vi "3Dlauncher.vi"(1 "dataFilePath":path, 2 "Data":string[][](array[string]), 3 "Template Filename":path, 4 "Channel Names":string[](array[string])) -> ()   [LabVIEW 2022 SP3]
uses:
  Anemometry/Anemometry Sub Vis/Controls/Group_Binning.ctl
  Anemometry/Anemometry Sub Vis/Data_plotting_vis/Results_plotter_Global.vi
panel:
  in  "Tab Control":enum32{"Page 1", "Page 2"}(tab)
  in  "Wind Direction":u16(ring) items=["Date Sortable", "Rig", "Run Command File", "Run Start Time", "Run Description", "Row Number", "Row Type", "Row Start (sec)", "Row Comment", "Timestamp", "Time In Row(s)", "Config", "Config Num", "Errata", "Omit", "WD", "WD.Pt", "WD.Pt.Cfg", "Point ID", "Point Row", "Legend0", "Downrange Distance (ft)", "Point Height Num", "Point Column", "Legend1", "- MeasuredVariables -----------", "-- VelocityStats --", "U_{dem} Nominal (m/s)", "U_{ref} (m/s)", "Uref ADAM (m/s)", "\\overline{U_{raw}} /U_{ref}", "U_{ref} ADAM /U_{ref}", "\\overline{U} (m/s)", "U corr (m/s)", "\\overline{V} (m/s)", "\\overline{W} (m/s)", "\\overline{|UV|} (m/s)", "\\overline{|UW|} (m/s)", "\\overline{|UVW|} (m/s)", "\\overline{\\theta} (deg)", "\\sigma^2(U) (m/s)^2", "\\sigma^2(V) (m/s)^2", "\\sigma^2(W) (m/s)^2", "\\sigma^2(|UV|) (m/s)^2", "\\sigma^2(|UW|) (m/s)^2", "\\sigma^2(|UVW|) (m/s)^2", "\\sigma^2(\\theta) (deg^2)", "u'v' (m^2/s^2)", "v'w' (m^2/s^2)", "u'w' (m^2/s^2)", "-- VelocityStatsEnd --", "-- QAstats --", "Omni meanPSU (V)", "Omni varPSU (V^2)", "Omni Cal Slope", "Omni Cal Intercept", "Temp (C)", "No Of Measurement Blocks", "No of Analogue Samples", "Flow Measurement Time", "Decimation", "AFRaw nGood perDecBlock", "AFGoodV nGood perDecBlock", "AFGoodVP nGood perDecBlock", "AFRaw nCone<58 deg", "AFRaw nCone<90 deg", "AFRaw Cone<58 deg", "AFRaw Cone<90 deg", "Run Messages", "-- QAstatsEnd --", "- MeasuredVariablesEnd -----------", "Max (ConeAngle) (deg)", "Valid AFReduction Fraction", "Valid Velocity Fraction", "Valid 5hpPressure Fraction", "- LocationsStart -------------", "Scale", "Probe Angle (deg)", "Row X 0", "X (mm)", "Y (mm)", "Z (mm)", "U_{ref} Z (mm)", "Metadata Motor X", "Metadata Motor Y", "Metadata Motor Z", "- LocationsEnd -------------", "- BLsetupBlock ------------", "BLS Trip[1] Ach(mm)", "BLS Trip[2] Ach(mm)", "BLS Spires[1] Ach(mm)", "BLS Spires[1]TipJoint Ach(mm)", "BLS Spires[1] Tips(mm)", "BLS Spires[2] Ach(mm)", "BLS Main[1] Ach(mm)", "BLS Main[2] Ach(mm)", "BLS Main[3] Ach(mm)", "BLS Boost[1] Ach(mm)", "BLS Boost[2] Ach(mm)", "BLS Boost[3] Ach(mm)", "Main Avg (mm)", "Boost Avg (mm)", "Spires[1] Total (mm)", "Ramp Request 0", "Ramp Request 1", "Ramp Request 2", "Ramp Request 3", "Ramp Request 4", "Ramp Request 5", "Ramp Request 6", "Ramp Request 7", "Ramp Request 8", "Ramp Request 9", "Ramp Request 10", "Ramp Request 11", "Ramp Request 12", "FORMATTED OUTPUT BELOW-THIS-------------", "Configuration", "Wind Direction (deg)", "BL Setup", "PointID", "Uref (m/s)", "Mean U /U_{ref}", "Mean V /U_{ref}", "Mean W /U_{ref}", "Mean |UV| /U_{ref}", "Mean |UW| /U_ref", "Mean |UVW| /U_ref", "Yaw (UV) (deg)", "TI (U) (/U)", "TI (U) (/|UV|)", "TI (V) (/|UV|)", "TI (W) (/|UW|)", "TI (|UV|) (/|UV|)", "TI (|UW|) (/|UW|)", "TI (|UVW|) (/|UVW|)", "TI Joint (%)", "Velocity Validation (percent)", "Raw Data Filename", "FORMATTED OUTPUT ABOVE-THIS---------------", "Current File", "Current Filepath", "Template File Used", "Seconds since 1st Jan", "Point Row Column", "Row Y", "X (in)", "Y (in)", "Z (in)", "STL name", "Coordinate System"]
  in  "STL":u16(ring) items=["Date Sortable", "Rig", "Run Command File", "Run Start Time", "Run Description", "Row Number", "Row Type", "Row Start (sec)", "Row Comment", "Timestamp", "Time In Row(s)", "Config", "Config Num", "Errata", "Omit", "WD", "WD.Pt", "WD.Pt.Cfg", "Point ID", "Point Row", "Legend0", "Downrange Distance (ft)", "Point Height Num", "Point Column", "Legend1", "- MeasuredVariables -----------", "-- VelocityStats --", "U_{dem} Nominal (m/s)", "U_{ref} (m/s)", "Uref ADAM (m/s)", "\\overline{U_{raw}} /U_{ref}", "U_{ref} ADAM /U_{ref}", "\\overline{U} (m/s)", "U corr (m/s)", "\\overline{V} (m/s)", "\\overline{W} (m/s)", "\\overline{|UV|} (m/s)", "\\overline{|UW|} (m/s)", "\\overline{|UVW|} (m/s)", "\\overline{\\theta} (deg)", "\\sigma^2(U) (m/s)^2", "\\sigma^2(V) (m/s)^2", "\\sigma^2(W) (m/s)^2", "\\sigma^2(|UV|) (m/s)^2", "\\sigma^2(|UW|) (m/s)^2", "\\sigma^2(|UVW|) (m/s)^2", "\\sigma^2(\\theta) (deg^2)", "u'v' (m^2/s^2)", "v'w' (m^2/s^2)", "u'w' (m^2/s^2)", "-- VelocityStatsEnd --", "-- QAstats --", "Omni meanPSU (V)", "Omni varPSU (V^2)", "Omni Cal Slope", "Omni Cal Intercept", "Temp (C)", "No Of Measurement Blocks", "No of Analogue Samples", "Flow Measurement Time", "Decimation", "AFRaw nGood perDecBlock", "AFGoodV nGood perDecBlock", "AFGoodVP nGood perDecBlock", "AFRaw nCone<58 deg", "AFRaw nCone<90 deg", "AFRaw Cone<58 deg", "AFRaw Cone<90 deg", "Run Messages", "-- QAstatsEnd --", "- MeasuredVariablesEnd -----------", "Max (ConeAngle) (deg)", "Valid AFReduction Fraction", "Valid Velocity Fraction", "Valid 5hpPressure Fraction", "- LocationsStart -------------", "Scale", "Probe Angle (deg)", "Row X 0", "X (mm)", "Y (mm)", "Z (mm)", "U_{ref} Z (mm)", "Metadata Motor X", "Metadata Motor Y", "Metadata Motor Z", "- LocationsEnd -------------", "- BLsetupBlock ------------", "BLS Trip[1] Ach(mm)", "BLS Trip[2] Ach(mm)", "BLS Spires[1] Ach(mm)", "BLS Spires[1]TipJoint Ach(mm)", "BLS Spires[1] Tips(mm)", "BLS Spires[2] Ach(mm)", "BLS Main[1] Ach(mm)", "BLS Main[2] Ach(mm)", "BLS Main[3] Ach(mm)", "BLS Boost[1] Ach(mm)", "BLS Boost[2] Ach(mm)", "BLS Boost[3] Ach(mm)", "Main Avg (mm)", "Boost Avg (mm)", "Spires[1] Total (mm)", "Ramp Request 0", "Ramp Request 1", "Ramp Request 2", "Ramp Request 3", "Ramp Request 4", "Ramp Request 5", "Ramp Request 6", "Ramp Request 7", "Ramp Request 8", "Ramp Request 9", "Ramp Request 10", "Ramp Request 11", "Ramp Request 12", "FORMATTED OUTPUT BELOW-THIS-------------", "Configuration", "Wind Direction (deg)", "BL Setup", "PointID", "Uref (m/s)", "Mean U /U_{ref}", "Mean V /U_{ref}", "Mean W /U_{ref}", "Mean |UV| /U_{ref}", "Mean |UW| /U_ref", "Mean |UVW| /U_ref", "Yaw (UV) (deg)", "TI (U) (/U)", "TI (U) (/|UV|)", "TI (V) (/|UV|)", "TI (W) (/|UW|)", "TI (|UV|) (/|UV|)", "TI (|UW|) (/|UW|)", "TI (|UVW|) (/|UVW|)", "TI Joint (%)", "Velocity Validation (percent)", "Raw Data Filename", "FORMATTED OUTPUT ABOVE-THIS---------------", "Current File", "Current Filepath", "Template File Used", "Seconds since 1st Jan", "Point Row Column", "Row Y", "X (in)", "Y (in)", "Z (in)", "STL name", "Coordinate System"]
  in  "OK Button":bool
  in  "vectorU":u16(ring) items=["Date Sortable", "Rig", "Run Command File", "Run Start Time", "Run Description", "Row Number", "Row Type", "Row Start (sec)", "Row Comment", "Timestamp", "Time In Row(s)", "Config", "Config Num", "Errata", "Omit", "WD", "WD.Pt", "WD.Pt.Cfg", "Point ID", "Point Row", "Legend0", "Downrange Distance (ft)", "Point Height Num", "Point Column", "Legend1", "- MeasuredVariables -----------", "-- VelocityStats --", "U_{dem} Nominal (m/s)", "U_{ref} (m/s)", "Uref ADAM (m/s)", "\\overline{U_{raw}} /U_{ref}", "U_{ref} ADAM /U_{ref}", "\\overline{U} (m/s)", "U corr (m/s)", "\\overline{V} (m/s)", "\\overline{W} (m/s)", "\\overline{|UV|} (m/s)", "\\overline{|UW|} (m/s)", "\\overline{|UVW|} (m/s)", "\\overline{\\theta} (deg)", "\\sigma^2(U) (m/s)^2", "\\sigma^2(V) (m/s)^2", "\\sigma^2(W) (m/s)^2", "\\sigma^2(|UV|) (m/s)^2", "\\sigma^2(|UW|) (m/s)^2", "\\sigma^2(|UVW|) (m/s)^2", "\\sigma^2(\\theta) (deg^2)", "u'v' (m^2/s^2)", "v'w' (m^2/s^2)", "u'w' (m^2/s^2)", "-- VelocityStatsEnd --", "-- QAstats --", "Omni meanPSU (V)", "Omni varPSU (V^2)", "Omni Cal Slope", "Omni Cal Intercept", "Temp (C)", "No Of Measurement Blocks", "No of Analogue Samples", "Flow Measurement Time", "Decimation", "AFRaw nGood perDecBlock", "AFGoodV nGood perDecBlock", "AFGoodVP nGood perDecBlock", "AFRaw nCone<58 deg", "AFRaw nCone<90 deg", "AFRaw Cone<58 deg", "AFRaw Cone<90 deg", "Run Messages", "-- QAstatsEnd --", "- MeasuredVariablesEnd -----------", "Max (ConeAngle) (deg)", "Valid AFReduction Fraction", "Valid Velocity Fraction", "Valid 5hpPressure Fraction", "- LocationsStart -------------", "Scale", "Probe Angle (deg)", "Row X 0", "X (mm)", "Y (mm)", "Z (mm)", "U_{ref} Z (mm)", "Metadata Motor X", "Metadata Motor Y", "Metadata Motor Z", "- LocationsEnd -------------", "- BLsetupBlock ------------", "BLS Trip[1] Ach(mm)", "BLS Trip[2] Ach(mm)", "BLS Spires[1] Ach(mm)", "BLS Spires[1]TipJoint Ach(mm)", "BLS Spires[1] Tips(mm)", "BLS Spires[2] Ach(mm)", "BLS Main[1] Ach(mm)", "BLS Main[2] Ach(mm)", "BLS Main[3] Ach(mm)", "BLS Boost[1] Ach(mm)", "BLS Boost[2] Ach(mm)", "BLS Boost[3] Ach(mm)", "Main Avg (mm)", "Boost Avg (mm)", "Spires[1] Total (mm)", "Ramp Request 0", "Ramp Request 1", "Ramp Request 2", "Ramp Request 3", "Ramp Request 4", "Ramp Request 5", "Ramp Request 6", "Ramp Request 7", "Ramp Request 8", "Ramp Request 9", "Ramp Request 10", "Ramp Request 11", "Ramp Request 12", "FORMATTED OUTPUT BELOW-THIS-------------", "Configuration", "Wind Direction (deg)", "BL Setup", "PointID", "Uref (m/s)", "Mean U /U_{ref}", "Mean V /U_{ref}", "Mean W /U_{ref}", "Mean |UV| /U_{ref}", "Mean |UW| /U_ref", "Mean |UVW| /U_ref", "Yaw (UV) (deg)", "TI (U) (/U)", "TI (U) (/|UV|)", "TI (V) (/|UV|)", "TI (W) (/|UW|)", "TI (|UV|) (/|UV|)", "TI (|UW|) (/|UW|)", "TI (|UVW|) (/|UVW|)", "TI Joint (%)", "Velocity Validation (percent)", "Raw Data Filename", "FORMATTED OUTPUT ABOVE-THIS---------------", "Current File", "Current Filepath", "Template File Used", "Seconds since 1st Jan", "Point Row Column", "Row Y", "X (in)", "Y (in)", "Z (in)", "STL name", "Coordinate System"]
  in  "vectorV":u16(ring) items=["Date Sortable", "Rig", "Run Command File", "Run Start Time", "Run Description", "Row Number", "Row Type", "Row Start (sec)", "Row Comment", "Timestamp", "Time In Row(s)", "Config", "Config Num", "Errata", "Omit", "WD", "WD.Pt", "WD.Pt.Cfg", "Point ID", "Point Row", "Legend0", "Downrange Distance (ft)", "Point Height Num", "Point Column", "Legend1", "- MeasuredVariables -----------", "-- VelocityStats --", "U_{dem} Nominal (m/s)", "U_{ref} (m/s)", "Uref ADAM (m/s)", "\\overline{U_{raw}} /U_{ref}", "U_{ref} ADAM /U_{ref}", "\\overline{U} (m/s)", "U corr (m/s)", "\\overline{V} (m/s)", "\\overline{W} (m/s)", "\\overline{|UV|} (m/s)", "\\overline{|UW|} (m/s)", "\\overline{|UVW|} (m/s)", "\\overline{\\theta} (deg)", "\\sigma^2(U) (m/s)^2", "\\sigma^2(V) (m/s)^2", "\\sigma^2(W) (m/s)^2", "\\sigma^2(|UV|) (m/s)^2", "\\sigma^2(|UW|) (m/s)^2", "\\sigma^2(|UVW|) (m/s)^2", "\\sigma^2(\\theta) (deg^2)", "u'v' (m^2/s^2)", "v'w' (m^2/s^2)", "u'w' (m^2/s^2)", "-- VelocityStatsEnd --", "-- QAstats --", "Omni meanPSU (V)", "Omni varPSU (V^2)", "Omni Cal Slope", "Omni Cal Intercept", "Temp (C)", "No Of Measurement Blocks", "No of Analogue Samples", "Flow Measurement Time", "Decimation", "AFRaw nGood perDecBlock", "AFGoodV nGood perDecBlock", "AFGoodVP nGood perDecBlock", "AFRaw nCone<58 deg", "AFRaw nCone<90 deg", "AFRaw Cone<58 deg", "AFRaw Cone<90 deg", "Run Messages", "-- QAstatsEnd --", "- MeasuredVariablesEnd -----------", "Max (ConeAngle) (deg)", "Valid AFReduction Fraction", "Valid Velocity Fraction", "Valid 5hpPressure Fraction", "- LocationsStart -------------", "Scale", "Probe Angle (deg)", "Row X 0", "X (mm)", "Y (mm)", "Z (mm)", "U_{ref} Z (mm)", "Metadata Motor X", "Metadata Motor Y", "Metadata Motor Z", "- LocationsEnd -------------", "- BLsetupBlock ------------", "BLS Trip[1] Ach(mm)", "BLS Trip[2] Ach(mm)", "BLS Spires[1] Ach(mm)", "BLS Spires[1]TipJoint Ach(mm)", "BLS Spires[1] Tips(mm)", "BLS Spires[2] Ach(mm)", "BLS Main[1] Ach(mm)", "BLS Main[2] Ach(mm)", "BLS Main[3] Ach(mm)", "BLS Boost[1] Ach(mm)", "BLS Boost[2] Ach(mm)", "BLS Boost[3] Ach(mm)", "Main Avg (mm)", "Boost Avg (mm)", "Spires[1] Total (mm)", "Ramp Request 0", "Ramp Request 1", "Ramp Request 2", "Ramp Request 3", "Ramp Request 4", "Ramp Request 5", "Ramp Request 6", "Ramp Request 7", "Ramp Request 8", "Ramp Request 9", "Ramp Request 10", "Ramp Request 11", "Ramp Request 12", "FORMATTED OUTPUT BELOW-THIS-------------", "Configuration", "Wind Direction (deg)", "BL Setup", "PointID", "Uref (m/s)", "Mean U /U_{ref}", "Mean V /U_{ref}", "Mean W /U_{ref}", "Mean |UV| /U_{ref}", "Mean |UW| /U_ref", "Mean |UVW| /U_ref", "Yaw (UV) (deg)", "TI (U) (/U)", "TI (U) (/|UV|)", "TI (V) (/|UV|)", "TI (W) (/|UW|)", "TI (|UV|) (/|UV|)", "TI (|UW|) (/|UW|)", "TI (|UVW|) (/|UVW|)", "TI Joint (%)", "Velocity Validation (percent)", "Raw Data Filename", "FORMATTED OUTPUT ABOVE-THIS---------------", "Current File", "Current Filepath", "Template File Used", "Seconds since 1st Jan", "Point Row Column", "Row Y", "X (in)", "Y (in)", "Z (in)", "STL name", "Coordinate System"]
  in  "vectorW":u16(ring) items=["Date Sortable", "Rig", "Run Command File", "Run Start Time", "Run Description", "Row Number", "Row Type", "Row Start (sec)", "Row Comment", "Timestamp", "Time In Row(s)", "Config", "Config Num", "Errata", "Omit", "WD", "WD.Pt", "WD.Pt.Cfg", "Point ID", "Point Row", "Legend0", "Downrange Distance (ft)", "Point Height Num", "Point Column", "Legend1", "- MeasuredVariables -----------", "-- VelocityStats --", "U_{dem} Nominal (m/s)", "U_{ref} (m/s)", "Uref ADAM (m/s)", "\\overline{U_{raw}} /U_{ref}", "U_{ref} ADAM /U_{ref}", "\\overline{U} (m/s)", "U corr (m/s)", "\\overline{V} (m/s)", "\\overline{W} (m/s)", "\\overline{|UV|} (m/s)", "\\overline{|UW|} (m/s)", "\\overline{|UVW|} (m/s)", "\\overline{\\theta} (deg)", "\\sigma^2(U) (m/s)^2", "\\sigma^2(V) (m/s)^2", "\\sigma^2(W) (m/s)^2", "\\sigma^2(|UV|) (m/s)^2", "\\sigma^2(|UW|) (m/s)^2", "\\sigma^2(|UVW|) (m/s)^2", "\\sigma^2(\\theta) (deg^2)", "u'v' (m^2/s^2)", "v'w' (m^2/s^2)", "u'w' (m^2/s^2)", "-- VelocityStatsEnd --", "-- QAstats --", "Omni meanPSU (V)", "Omni varPSU (V^2)", "Omni Cal Slope", "Omni Cal Intercept", "Temp (C)", "No Of Measurement Blocks", "No of Analogue Samples", "Flow Measurement Time", "Decimation", "AFRaw nGood perDecBlock", "AFGoodV nGood perDecBlock", "AFGoodVP nGood perDecBlock", "AFRaw nCone<58 deg", "AFRaw nCone<90 deg", "AFRaw Cone<58 deg", "AFRaw Cone<90 deg", "Run Messages", "-- QAstatsEnd --", "- MeasuredVariablesEnd -----------", "Max (ConeAngle) (deg)", "Valid AFReduction Fraction", "Valid Velocity Fraction", "Valid 5hpPressure Fraction", "- LocationsStart -------------", "Scale", "Probe Angle (deg)", "Row X 0", "X (mm)", "Y (mm)", "Z (mm)", "U_{ref} Z (mm)", "Metadata Motor X", "Metadata Motor Y", "Metadata Motor Z", "- LocationsEnd -------------", "- BLsetupBlock ------------", "BLS Trip[1] Ach(mm)", "BLS Trip[2] Ach(mm)", "BLS Spires[1] Ach(mm)", "BLS Spires[1]TipJoint Ach(mm)", "BLS Spires[1] Tips(mm)", "BLS Spires[2] Ach(mm)", "BLS Main[1] Ach(mm)", "BLS Main[2] Ach(mm)", "BLS Main[3] Ach(mm)", "BLS Boost[1] Ach(mm)", "BLS Boost[2] Ach(mm)", "BLS Boost[3] Ach(mm)", "Main Avg (mm)", "Boost Avg (mm)", "Spires[1] Total (mm)", "Ramp Request 0", "Ramp Request 1", "Ramp Request 2", "Ramp Request 3", "Ramp Request 4", "Ramp Request 5", "Ramp Request 6", "Ramp Request 7", "Ramp Request 8", "Ramp Request 9", "Ramp Request 10", "Ramp Request 11", "Ramp Request 12", "FORMATTED OUTPUT BELOW-THIS-------------", "Configuration", "Wind Direction (deg)", "BL Setup", "PointID", "Uref (m/s)", "Mean U /U_{ref}", "Mean V /U_{ref}", "Mean W /U_{ref}", "Mean |UV| /U_{ref}", "Mean |UW| /U_ref", "Mean |UVW| /U_ref", "Yaw (UV) (deg)", "TI (U) (/U)", "TI (U) (/|UV|)", "TI (V) (/|UV|)", "TI (W) (/|UW|)", "TI (|UV|) (/|UV|)", "TI (|UW|) (/|UW|)", "TI (|UVW|) (/|UVW|)", "TI Joint (%)", "Velocity Validation (percent)", "Raw Data Filename", "FORMATTED OUTPUT ABOVE-THIS---------------", "Current File", "Current Filepath", "Template File Used", "Seconds since 1st Jan", "Point Row Column", "Row Y", "X (in)", "Y (in)", "Z (in)", "STL name", "Coordinate System"]
  in  "Scalar":u16(ring) items=["Date Sortable", "Rig", "Run Command File", "Run Start Time", "Run Description", "Row Number", "Row Type", "Row Start (sec)", "Row Comment", "Timestamp", "Time In Row(s)", "Config", "Config Num", "Errata", "Omit", "WD", "WD.Pt", "WD.Pt.Cfg", "Point ID", "Point Row", "Legend0", "Downrange Distance (ft)", "Point Height Num", "Point Column", "Legend1", "- MeasuredVariables -----------", "-- VelocityStats --", "U_{dem} Nominal (m/s)", "U_{ref} (m/s)", "Uref ADAM (m/s)", "\\overline{U_{raw}} /U_{ref}", "U_{ref} ADAM /U_{ref}", "\\overline{U} (m/s)", "U corr (m/s)", "\\overline{V} (m/s)", "\\overline{W} (m/s)", "\\overline{|UV|} (m/s)", "\\overline{|UW|} (m/s)", "\\overline{|UVW|} (m/s)", "\\overline{\\theta} (deg)", "\\sigma^2(U) (m/s)^2", "\\sigma^2(V) (m/s)^2", "\\sigma^2(W) (m/s)^2", "\\sigma^2(|UV|) (m/s)^2", "\\sigma^2(|UW|) (m/s)^2", "\\sigma^2(|UVW|) (m/s)^2", "\\sigma^2(\\theta) (deg^2)", "u'v' (m^2/s^2)", "v'w' (m^2/s^2)", "u'w' (m^2/s^2)", "-- VelocityStatsEnd --", "-- QAstats --", "Omni meanPSU (V)", "Omni varPSU (V^2)", "Omni Cal Slope", "Omni Cal Intercept", "Temp (C)", "No Of Measurement Blocks", "No of Analogue Samples", "Flow Measurement Time", "Decimation", "AFRaw nGood perDecBlock", "AFGoodV nGood perDecBlock", "AFGoodVP nGood perDecBlock", "AFRaw nCone<58 deg", "AFRaw nCone<90 deg", "AFRaw Cone<58 deg", "AFRaw Cone<90 deg", "Run Messages", "-- QAstatsEnd --", "- MeasuredVariablesEnd -----------", "Max (ConeAngle) (deg)", "Valid AFReduction Fraction", "Valid Velocity Fraction", "Valid 5hpPressure Fraction", "- LocationsStart -------------", "Scale", "Probe Angle (deg)", "Row X 0", "X (mm)", "Y (mm)", "Z (mm)", "U_{ref} Z (mm)", "Metadata Motor X", "Metadata Motor Y", "Metadata Motor Z", "- LocationsEnd -------------", "- BLsetupBlock ------------", "BLS Trip[1] Ach(mm)", "BLS Trip[2] Ach(mm)", "BLS Spires[1] Ach(mm)", "BLS Spires[1]TipJoint Ach(mm)", "BLS Spires[1] Tips(mm)", "BLS Spires[2] Ach(mm)", "BLS Main[1] Ach(mm)", "BLS Main[2] Ach(mm)", "BLS Main[3] Ach(mm)", "BLS Boost[1] Ach(mm)", "BLS Boost[2] Ach(mm)", "BLS Boost[3] Ach(mm)", "Main Avg (mm)", "Boost Avg (mm)", "Spires[1] Total (mm)", "Ramp Request 0", "Ramp Request 1", "Ramp Request 2", "Ramp Request 3", "Ramp Request 4", "Ramp Request 5", "Ramp Request 6", "Ramp Request 7", "Ramp Request 8", "Ramp Request 9", "Ramp Request 10", "Ramp Request 11", "Ramp Request 12", "FORMATTED OUTPUT BELOW-THIS-------------", "Configuration", "Wind Direction (deg)", "BL Setup", "PointID", "Uref (m/s)", "Mean U /U_{ref}", "Mean V /U_{ref}", "Mean W /U_{ref}", "Mean |UV| /U_{ref}", "Mean |UW| /U_ref", "Mean |UVW| /U_ref", "Yaw (UV) (deg)", "TI (U) (/U)", "TI (U) (/|UV|)", "TI (V) (/|UV|)", "TI (W) (/|UW|)", "TI (|UV|) (/|UV|)", "TI (|UW|) (/|UW|)", "TI (|UVW|) (/|UVW|)", "TI Joint (%)", "Velocity Validation (percent)", "Raw Data Filename", "FORMATTED OUTPUT ABOVE-THIS---------------", "Current File", "Current Filepath", "Template File Used", "Seconds since 1st Jan", "Point Row Column", "Row Y", "X (in)", "Y (in)", "Z (in)", "STL name", "Coordinate System"]
  in  "Location X":u16(ring) items=["Date Sortable", "Rig", "Run Command File", "Run Start Time", "Run Description", "Row Number", "Row Type", "Row Start (sec)", "Row Comment", "Timestamp", "Time In Row(s)", "Config", "Config Num", "Errata", "Omit", "WD", "WD.Pt", "WD.Pt.Cfg", "Point ID", "Point Row", "Legend0", "Downrange Distance (ft)", "Point Height Num", "Point Column", "Legend1", "- MeasuredVariables -----------", "-- VelocityStats --", "U_{dem} Nominal (m/s)", "U_{ref} (m/s)", "Uref ADAM (m/s)", "\\overline{U_{raw}} /U_{ref}", "U_{ref} ADAM /U_{ref}", "\\overline{U} (m/s)", "U corr (m/s)", "\\overline{V} (m/s)", "\\overline{W} (m/s)", "\\overline{|UV|} (m/s)", "\\overline{|UW|} (m/s)", "\\overline{|UVW|} (m/s)", "\\overline{\\theta} (deg)", "\\sigma^2(U) (m/s)^2", "\\sigma^2(V) (m/s)^2", "\\sigma^2(W) (m/s)^2", "\\sigma^2(|UV|) (m/s)^2", "\\sigma^2(|UW|) (m/s)^2", "\\sigma^2(|UVW|) (m/s)^2", "\\sigma^2(\\theta) (deg^2)", "u'v' (m^2/s^2)", "v'w' (m^2/s^2)", "u'w' (m^2/s^2)", "-- VelocityStatsEnd --", "-- QAstats --", "Omni meanPSU (V)", "Omni varPSU (V^2)", "Omni Cal Slope", "Omni Cal Intercept", "Temp (C)", "No Of Measurement Blocks", "No of Analogue Samples", "Flow Measurement Time", "Decimation", "AFRaw nGood perDecBlock", "AFGoodV nGood perDecBlock", "AFGoodVP nGood perDecBlock", "AFRaw nCone<58 deg", "AFRaw nCone<90 deg", "AFRaw Cone<58 deg", "AFRaw Cone<90 deg", "Run Messages", "-- QAstatsEnd --", "- MeasuredVariablesEnd -----------", "Max (ConeAngle) (deg)", "Valid AFReduction Fraction", "Valid Velocity Fraction", "Valid 5hpPressure Fraction", "- LocationsStart -------------", "Scale", "Probe Angle (deg)", "Row X 0", "X (mm)", "Y (mm)", "Z (mm)", "U_{ref} Z (mm)", "Metadata Motor X", "Metadata Motor Y", "Metadata Motor Z", "- LocationsEnd -------------", "- BLsetupBlock ------------", "BLS Trip[1] Ach(mm)", "BLS Trip[2] Ach(mm)", "BLS Spires[1] Ach(mm)", "BLS Spires[1]TipJoint Ach(mm)", "BLS Spires[1] Tips(mm)", "BLS Spires[2] Ach(mm)", "BLS Main[1] Ach(mm)", "BLS Main[2] Ach(mm)", "BLS Main[3] Ach(mm)", "BLS Boost[1] Ach(mm)", "BLS Boost[2] Ach(mm)", "BLS Boost[3] Ach(mm)", "Main Avg (mm)", "Boost Avg (mm)", "Spires[1] Total (mm)", "Ramp Request 0", "Ramp Request 1", "Ramp Request 2", "Ramp Request 3", "Ramp Request 4", "Ramp Request 5", "Ramp Request 6", "Ramp Request 7", "Ramp Request 8", "Ramp Request 9", "Ramp Request 10", "Ramp Request 11", "Ramp Request 12", "FORMATTED OUTPUT BELOW-THIS-------------", "Configuration", "Wind Direction (deg)", "BL Setup", "PointID", "Uref (m/s)", "Mean U /U_{ref}", "Mean V /U_{ref}", "Mean W /U_{ref}", "Mean |UV| /U_{ref}", "Mean |UW| /U_ref", "Mean |UVW| /U_ref", "Yaw (UV) (deg)", "TI (U) (/U)", "TI (U) (/|UV|)", "TI (V) (/|UV|)", "TI (W) (/|UW|)", "TI (|UV|) (/|UV|)", "TI (|UW|) (/|UW|)", "TI (|UVW|) (/|UVW|)", "TI Joint (%)", "Velocity Validation (percent)", "Raw Data Filename", "FORMATTED OUTPUT ABOVE-THIS---------------", "Current File", "Current Filepath", "Template File Used", "Seconds since 1st Jan", "Point Row Column", "Row Y", "X (in)", "Y (in)", "Z (in)", "STL name", "Coordinate System"]
  in  "Location Y":u16(ring) items=["Date Sortable", "Rig", "Run Command File", "Run Start Time", "Run Description", "Row Number", "Row Type", "Row Start (sec)", "Row Comment", "Timestamp", "Time In Row(s)", "Config", "Config Num", "Errata", "Omit", "WD", "WD.Pt", "WD.Pt.Cfg", "Point ID", "Point Row", "Legend0", "Downrange Distance (ft)", "Point Height Num", "Point Column", "Legend1", "- MeasuredVariables -----------", "-- VelocityStats --", "U_{dem} Nominal (m/s)", "U_{ref} (m/s)", "Uref ADAM (m/s)", "\\overline{U_{raw}} /U_{ref}", "U_{ref} ADAM /U_{ref}", "\\overline{U} (m/s)", "U corr (m/s)", "\\overline{V} (m/s)", "\\overline{W} (m/s)", "\\overline{|UV|} (m/s)", "\\overline{|UW|} (m/s)", "\\overline{|UVW|} (m/s)", "\\overline{\\theta} (deg)", "\\sigma^2(U) (m/s)^2", "\\sigma^2(V) (m/s)^2", "\\sigma^2(W) (m/s)^2", "\\sigma^2(|UV|) (m/s)^2", "\\sigma^2(|UW|) (m/s)^2", "\\sigma^2(|UVW|) (m/s)^2", "\\sigma^2(\\theta) (deg^2)", "u'v' (m^2/s^2)", "v'w' (m^2/s^2)", "u'w' (m^2/s^2)", "-- VelocityStatsEnd --", "-- QAstats --", "Omni meanPSU (V)", "Omni varPSU (V^2)", "Omni Cal Slope", "Omni Cal Intercept", "Temp (C)", "No Of Measurement Blocks", "No of Analogue Samples", "Flow Measurement Time", "Decimation", "AFRaw nGood perDecBlock", "AFGoodV nGood perDecBlock", "AFGoodVP nGood perDecBlock", "AFRaw nCone<58 deg", "AFRaw nCone<90 deg", "AFRaw Cone<58 deg", "AFRaw Cone<90 deg", "Run Messages", "-- QAstatsEnd --", "- MeasuredVariablesEnd -----------", "Max (ConeAngle) (deg)", "Valid AFReduction Fraction", "Valid Velocity Fraction", "Valid 5hpPressure Fraction", "- LocationsStart -------------", "Scale", "Probe Angle (deg)", "Row X 0", "X (mm)", "Y (mm)", "Z (mm)", "U_{ref} Z (mm)", "Metadata Motor X", "Metadata Motor Y", "Metadata Motor Z", "- LocationsEnd -------------", "- BLsetupBlock ------------", "BLS Trip[1] Ach(mm)", "BLS Trip[2] Ach(mm)", "BLS Spires[1] Ach(mm)", "BLS Spires[1]TipJoint Ach(mm)", "BLS Spires[1] Tips(mm)", "BLS Spires[2] Ach(mm)", "BLS Main[1] Ach(mm)", "BLS Main[2] Ach(mm)", "BLS Main[3] Ach(mm)", "BLS Boost[1] Ach(mm)", "BLS Boost[2] Ach(mm)", "BLS Boost[3] Ach(mm)", "Main Avg (mm)", "Boost Avg (mm)", "Spires[1] Total (mm)", "Ramp Request 0", "Ramp Request 1", "Ramp Request 2", "Ramp Request 3", "Ramp Request 4", "Ramp Request 5", "Ramp Request 6", "Ramp Request 7", "Ramp Request 8", "Ramp Request 9", "Ramp Request 10", "Ramp Request 11", "Ramp Request 12", "FORMATTED OUTPUT BELOW-THIS-------------", "Configuration", "Wind Direction (deg)", "BL Setup", "PointID", "Uref (m/s)", "Mean U /U_{ref}", "Mean V /U_{ref}", "Mean W /U_{ref}", "Mean |UV| /U_{ref}", "Mean |UW| /U_ref", "Mean |UVW| /U_ref", "Yaw (UV) (deg)", "TI (U) (/U)", "TI (U) (/|UV|)", "TI (V) (/|UV|)", "TI (W) (/|UW|)", "TI (|UV|) (/|UV|)", "TI (|UW|) (/|UW|)", "TI (|UVW|) (/|UVW|)", "TI Joint (%)", "Velocity Validation (percent)", "Raw Data Filename", "FORMATTED OUTPUT ABOVE-THIS---------------", "Current File", "Current Filepath", "Template File Used", "Seconds since 1st Jan", "Point Row Column", "Row Y", "X (in)", "Y (in)", "Z (in)", "STL name", "Coordinate System"]
  in  "Location Z":u16(ring) items=["Date Sortable", "Rig", "Run Command File", "Run Start Time", "Run Description", "Row Number", "Row Type", "Row Start (sec)", "Row Comment", "Timestamp", "Time In Row(s)", "Config", "Config Num", "Errata", "Omit", "WD", "WD.Pt", "WD.Pt.Cfg", "Point ID", "Point Row", "Legend0", "Downrange Distance (ft)", "Point Height Num", "Point Column", "Legend1", "- MeasuredVariables -----------", "-- VelocityStats --", "U_{dem} Nominal (m/s)", "U_{ref} (m/s)", "Uref ADAM (m/s)", "\\overline{U_{raw}} /U_{ref}", "U_{ref} ADAM /U_{ref}", "\\overline{U} (m/s)", "U corr (m/s)", "\\overline{V} (m/s)", "\\overline{W} (m/s)", "\\overline{|UV|} (m/s)", "\\overline{|UW|} (m/s)", "\\overline{|UVW|} (m/s)", "\\overline{\\theta} (deg)", "\\sigma^2(U) (m/s)^2", "\\sigma^2(V) (m/s)^2", "\\sigma^2(W) (m/s)^2", "\\sigma^2(|UV|) (m/s)^2", "\\sigma^2(|UW|) (m/s)^2", "\\sigma^2(|UVW|) (m/s)^2", "\\sigma^2(\\theta) (deg^2)", "u'v' (m^2/s^2)", "v'w' (m^2/s^2)", "u'w' (m^2/s^2)", "-- VelocityStatsEnd --", "-- QAstats --", "Omni meanPSU (V)", "Omni varPSU (V^2)", "Omni Cal Slope", "Omni Cal Intercept", "Temp (C)", "No Of Measurement Blocks", "No of Analogue Samples", "Flow Measurement Time", "Decimation", "AFRaw nGood perDecBlock", "AFGoodV nGood perDecBlock", "AFGoodVP nGood perDecBlock", "AFRaw nCone<58 deg", "AFRaw nCone<90 deg", "AFRaw Cone<58 deg", "AFRaw Cone<90 deg", "Run Messages", "-- QAstatsEnd --", "- MeasuredVariablesEnd -----------", "Max (ConeAngle) (deg)", "Valid AFReduction Fraction", "Valid Velocity Fraction", "Valid 5hpPressure Fraction", "- LocationsStart -------------", "Scale", "Probe Angle (deg)", "Row X 0", "X (mm)", "Y (mm)", "Z (mm)", "U_{ref} Z (mm)", "Metadata Motor X", "Metadata Motor Y", "Metadata Motor Z", "- LocationsEnd -------------", "- BLsetupBlock ------------", "BLS Trip[1] Ach(mm)", "BLS Trip[2] Ach(mm)", "BLS Spires[1] Ach(mm)", "BLS Spires[1]TipJoint Ach(mm)", "BLS Spires[1] Tips(mm)", "BLS Spires[2] Ach(mm)", "BLS Main[1] Ach(mm)", "BLS Main[2] Ach(mm)", "BLS Main[3] Ach(mm)", "BLS Boost[1] Ach(mm)", "BLS Boost[2] Ach(mm)", "BLS Boost[3] Ach(mm)", "Main Avg (mm)", "Boost Avg (mm)", "Spires[1] Total (mm)", "Ramp Request 0", "Ramp Request 1", "Ramp Request 2", "Ramp Request 3", "Ramp Request 4", "Ramp Request 5", "Ramp Request 6", "Ramp Request 7", "Ramp Request 8", "Ramp Request 9", "Ramp Request 10", "Ramp Request 11", "Ramp Request 12", "FORMATTED OUTPUT BELOW-THIS-------------", "Configuration", "Wind Direction (deg)", "BL Setup", "PointID", "Uref (m/s)", "Mean U /U_{ref}", "Mean V /U_{ref}", "Mean W /U_{ref}", "Mean |UV| /U_{ref}", "Mean |UW| /U_ref", "Mean |UVW| /U_ref", "Yaw (UV) (deg)", "TI (U) (/U)", "TI (U) (/|UV|)", "TI (V) (/|UV|)", "TI (W) (/|UW|)", "TI (|UV|) (/|UV|)", "TI (|UW|) (/|UW|)", "TI (|UVW|) (/|UVW|)", "TI Joint (%)", "Velocity Validation (percent)", "Raw Data Filename", "FORMATTED OUTPUT ABOVE-THIS---------------", "Current File", "Current Filepath", "Template File Used", "Seconds since 1st Jan", "Point Row Column", "Row Y", "X (in)", "Y (in)", "Z (in)", "STL name", "Coordinate System"]
  out "dataFilePathOut":path
  in  "Row Selector":i32(listbox)=1
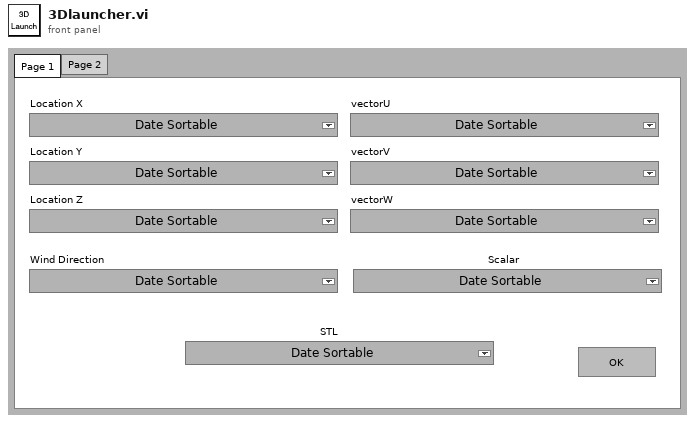
[diagram p1: front panel]
types:
  T1 = enum16{"Show only data summary", "Show data summary", "No data summary"}
  T2 = typedef "Group_Binning.ctl" = cluster{"Index":i32, "Tolerance":dbl, "Precision":string}
  T3 = enum32{"Invalid", "Standard", "Closed", "Hidden", "Minimized", "Maximized"}
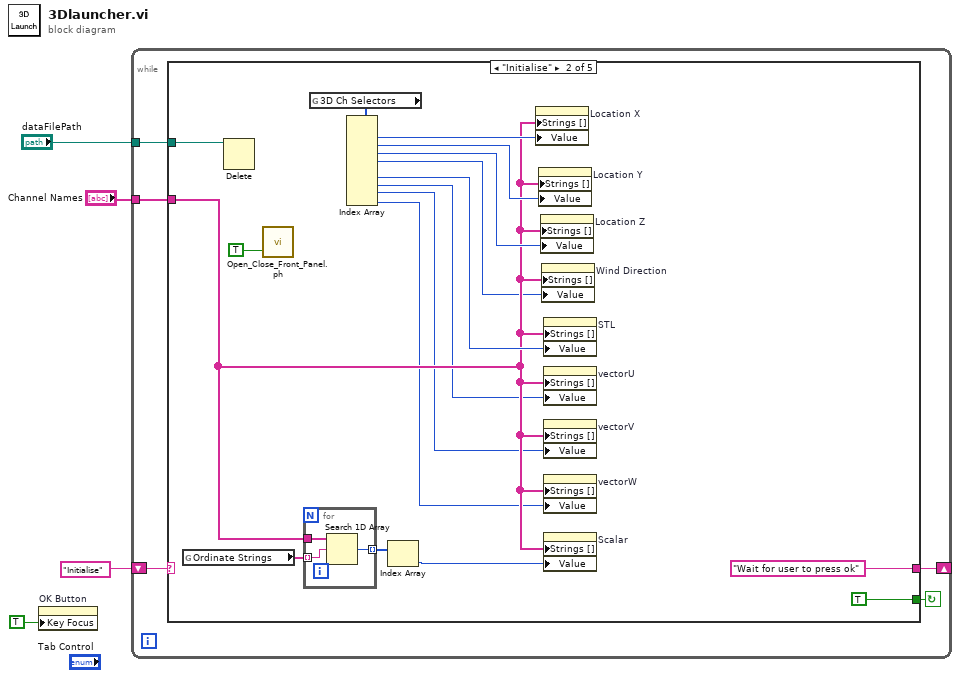
[diagram p0: block diagram]
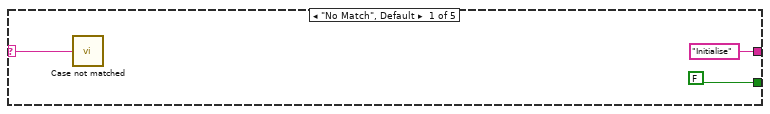
[diagram p2: hidden frame]
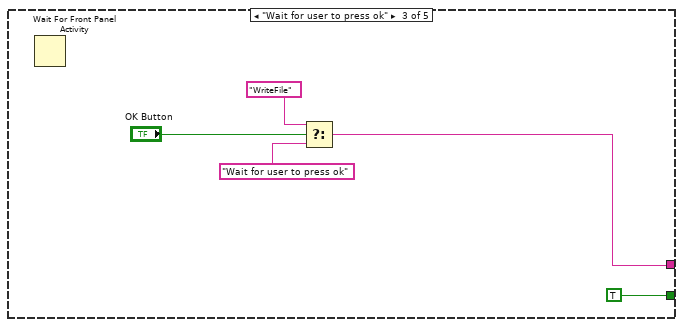
[diagram p3: hidden frame]
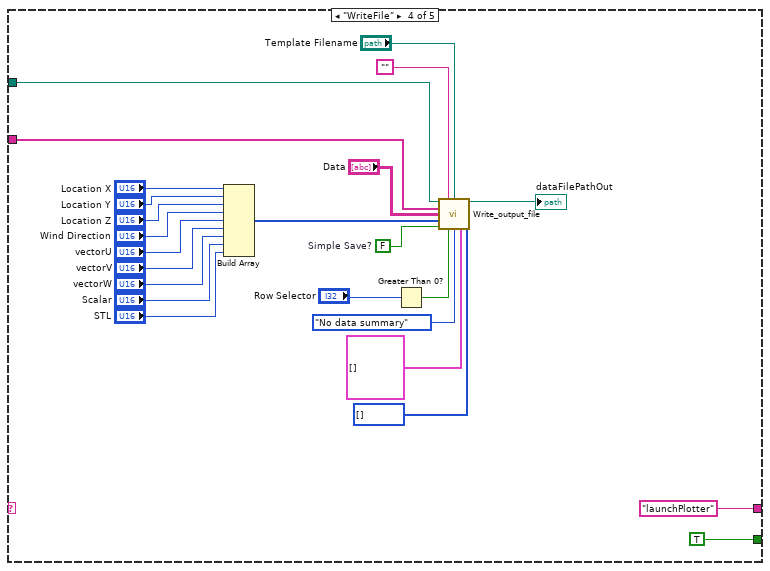
[diagram p4: hidden frame]
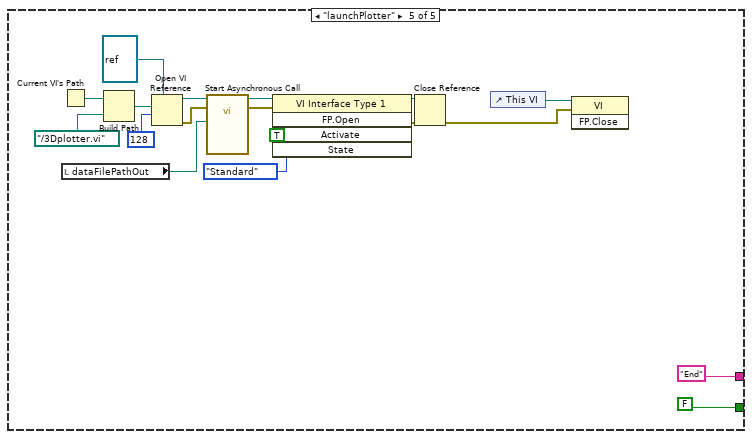
[diagram p5: hidden frame]
diagram:
  n1 = property on="OK Button" class="Bool"("Key Focus"=TRUE) -> ()  [unwired: 2 in, 2 out]
  n2 = while {
    shift-left: "Initialise" -> [w7]
    shift-right: [w8] -> _
    tunnel: "Channel Names" -> [w6]
    tunnel: "dataFilePath" -> [w5]
    stop <- w9 continue-if-true
    n3 = case shown="\"Initialise\"" w7 {
      selector: w7 -> [w10 _ _ _ _]
      tunnel: [FALSE TRUE TRUE TRUE FALSE] -> w9
      tunnel: ["Initialise" "Wait for user to press ok" w36 "launchPlotter" ("t") "End" ("t")] -> w8
      tunnel: w6 -> [_ w18 _ w43 _]
      tunnel: w5 -> [_ w26 _ w51 _]
      frame "No Match", Default {
        n4 = call "Case not matched.vi"("Case Name not Matched"=w10) -> ()
      }
      frame "Initialise" {
        n5 = global read "Results_plotter_Global.vi" "Ordinate Strings"() -> (w20:string[])
        n6 = Delete(path (use dialog)=w26) -> ()  [unwired: 1 in, 6 out]
        n7 = call "Open_Close_Front_Panel.ph.vi"("openWindow (T)"=TRUE ("Front Panel Window:Open")) -> ()  [unwired: 2 in, 1 out]
        n8 = for {
          tunnel: w18 -> [w32]
          tunnel: w20 -> [w31] mode=indexing
          tunnel: [w30] -> w19 mode=indexing
          n9 = Search 1D Array(1D array=w32, element=w31) -> (index of element=w30:i32)  [unwired: 1 in]
        }
        n10 = global read "Results_plotter_Global.vi" "3D Ch Selectors"() -> (w25:i32[])
        n11 = Index Array(array=w25) -> (element #1=w24:i32, element #2=w23:i32, element #3=w22:i32, element #4=w17:i32, element #6=w21:i32, element #7=w15:i32, element #8=w14:i32, element #9=w13:i32)  [unwired: 9 in, 1 out]
        n12 = Index Array(array=w19) -> (element=w16:i32)  [unwired: 1 in]
        n13 = property on="Location X" class="Ring (strict)"("Strings []"=w18, "Value"=w24) -> ()  [unwired: 2 in, 2 out]
        n14 = property on="Location Y" class="Ring (strict)"("Strings []"=w18, "Value"=w23) -> ()  [unwired: 2 in, 2 out]
        n15 = property on="Location Z" class="Ring (strict)"("Strings []"=w18, "Value"=w22) -> ()  [unwired: 2 in, 2 out]
        n16 = property on="Wind Direction" class="Ring (strict)"("Strings []"=w18, "Value"=w17) -> ()  [unwired: 2 in, 2 out]
        n17 = property on="STL" class="Ring (strict)"("Strings []"=w18, "Value"=w21) -> ()  [unwired: 2 in, 2 out]
        n18 = property on="vectorU" class="Ring (strict)"("Strings []"=w18, "Value"=w15) -> ()  [unwired: 2 in, 2 out]
        n19 = property on="vectorV" class="Ring (strict)"("Strings []"=w18, "Value"=w14) -> ()  [unwired: 2 in, 2 out]
        n20 = property on="vectorW" class="Ring (strict)"("Strings []"=w18, "Value"=w13) -> ()  [unwired: 2 in, 2 out]
        n21 = property on="Scalar" class="Ring (strict)"("Strings []"=w18, "Value"=w16) -> ()  [unwired: 2 in, 2 out]
      }
      frame "Wait for user to press ok" {
        n22 = Wait For Front Panel Activity() -> ()  [unwired: 3 in, 1 out]
        n23 = Select(t="WriteFile", s="OK Button", f="Wait for user to press ok") -> (s? t:f=w36:string)
      }
      frame "WriteFile" {
        w42 = FALSE  # Simple Save?
        n24 = Build Array("Location X", "Location Y", "Location Z", "Wind Direction", "vectorU", "vectorV", "vectorW", "Scalar", "STL") -> (w44:u16[])
        n25 = Greater Than 0?(x="Row Selector") -> (x > 0?=w55:bool)
        n26 = call "Write_output_file.vi"("Output filename"=w51, "Header"="", "Template Filename"="Template Filename", "Channel Names"=w43, "Data"="Data", "Desired Columns"=w44, "Simple Save?"=w42, "Save Plotted rows only?"=w55, "Summarise mode"=T1."No data summary", "Grouping info"=T2[] [], "Channels to Tabulate in header"=i32[] []) -> ("Output filename Out"=→"dataFilePathOut":path)  [unwired: 1 in, 3 out]
      }
      frame "launchPlotter" {
        n27 = Current VI's Path() -> (path=w74:path)
        n28 = local read "dataFilePathOut"() -> (w62:path)
        n29 = Build Path(base path=w74, name or relative path=path "../3Dplotter.vi") -> (appended path=w73:path)
        n30 = Open VI Reference(type specifier VI Refnum (for type only)=refnum<vi> refnum, vi path=w73, options=128) -> (vi reference=w72:refnum<vi>, error out=w71:errorcluster)  [unwired: 3 in]
        n31 = call-by-ref "Start Asynchronous Call"(reference=w72, error in=w71, "vectorFile1"=w62) -> (reference out=w70:refnum<vi>, error out=w75:errorcluster)  [unwired: 11 in]
        n32 = invoke class="VI Interface Type 1" method="FP.Open"(reference=w70, error in=w75, "Activate"=TRUE ("Activate?"), "State"=T3."Standard") -> (reference out=w76:refnum<vi>, error out=w77:errorcluster)  [unwired: 1 in, 3 out]
        n33 = Close Reference(reference=w76, error in (no error)=w77) -> (error out=w63:errorcluster)
        n34 = control-ref of="This VI"() -> (w64:refnum<vi>)
        n35 = invoke class="VI" method="FP.Close"(reference=w64, error in=w63) -> ()  [unwired: 1 in, 3 out]
      }
    }
  }
